vi "drawchart.vi"() -> ()   [LabVIEW 2012]
uses:
  <vilib>/Utility/miscctls.llb/LVDateTimeRec.ctl
  <vilib>/addons/database/Auxilliary.llb/DB Tools Cursor Type.ctl
  <vilib>/addons/database/Connection.llb/DB Tools Open Connec (Path).vi
  <vilib>/addons/database/Connection.llb/Conn Execute.vi
  <vilib>/addons/database/Recordset.llb/Rec Destroy - Connection.vi
  <vilib>/addons/database/_DB Variant To Data/Database Variant To Data.xnode
  <vilib>/addons/database/NI_Database_API.lvlib
panel:
  out "Waveform Graph":i32[](graph)
  out "Array":i32[](array[numeric])
  out "error out":errorcluster
  in  "Cluster":cluster{"rep_date":string, "rep_val":dbl}
  in  "date time rec":T1
  in  "beg_date":string
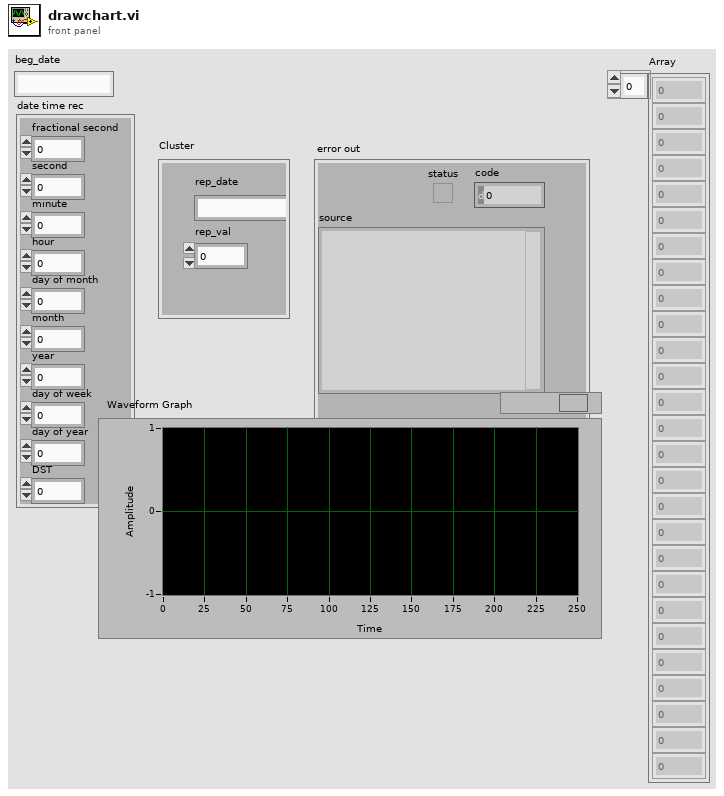
[diagram p1: front panel]
types:
  T1 = typedef "LVDateTimeRec.ctl" = cluster{"fractional second":dbl, "second":i32, "minute":i32, "hour":i32, "day of month":i32, "month":i32, "year":i32, "day of week":i32, "day of year":i32, "DST":i32}
  T2 = typedef "NI_Database_API.lvlib/Conn ObjectReference.ctl" = refnum<k1>
  T3 = typedef "NI_Database_API.lvlib/DB Tools Cursor Type.ctl" = enum16{"forward-only", "keyset", "dynamic", "static"}
  T4 = typedef "NI_Database_API.lvlib/Rec ObjectReference.ctl" = refnum<k1>
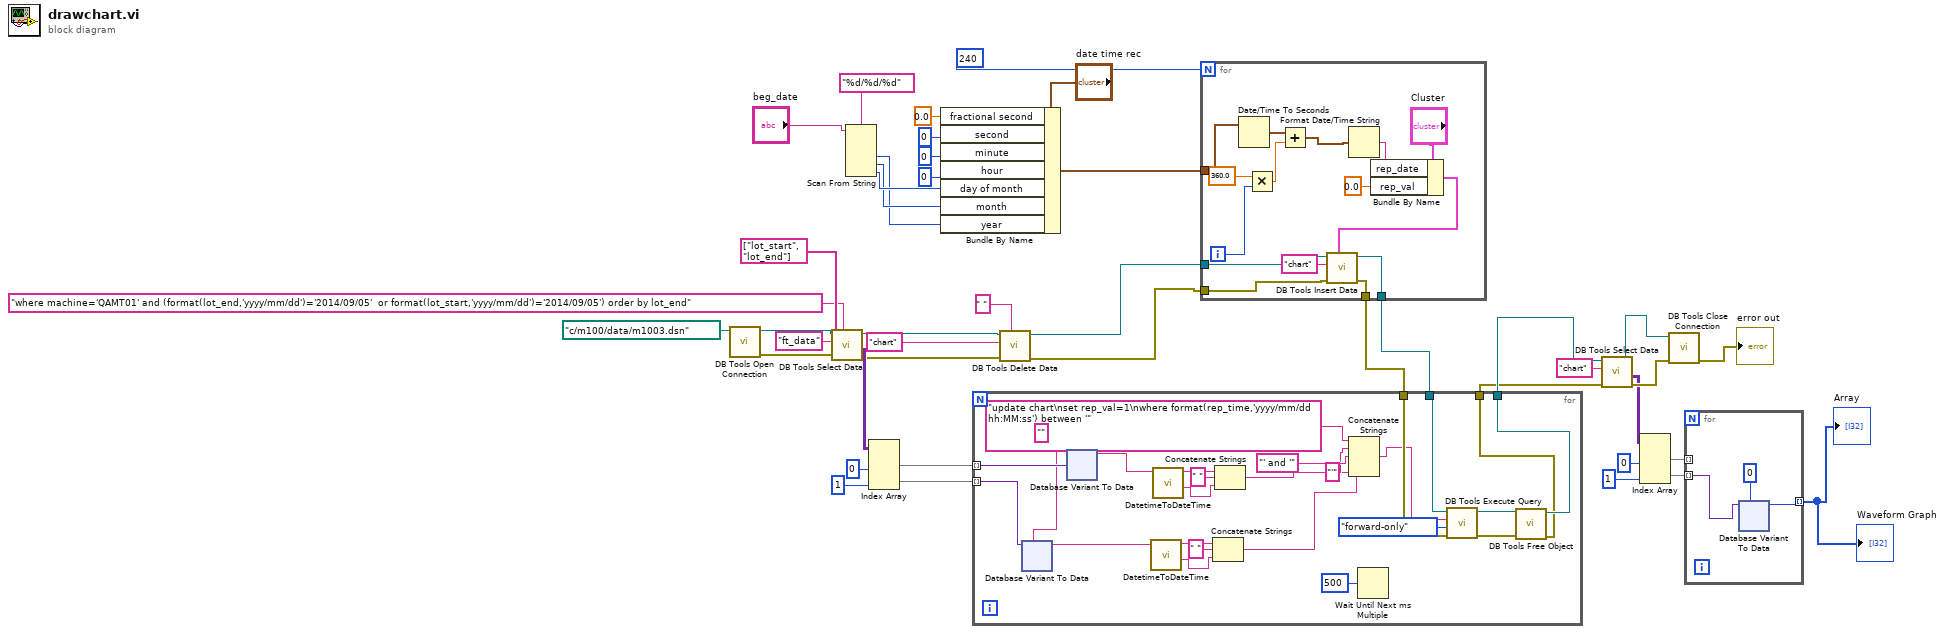
[diagram p0: block diagram]
diagram:
  n1 = call-poly <vilib>:"DB Tools Open Connection.vi"("connection information"=path "c:/m100/data/m1003.dsn") -> ("error out"=w41:errorcluster, "connection reference"=w42:T2)  [unwired: 7 in]
  n2 = call <vilib>:"DB Tools Select Data.vi"("condition"="where machine='QAMT01' and (format(lot_end,'yyyy/mm/dd')='2014/09/05'  or format(lot_start,'yyyy/mm/dd')='2014/09/05') order by lot_end", "error in (no error)"=w41, "columns"=string[] ["lot_start", "lot_end"], "table"="ft_data", "connection reference"=w42) -> ("error out"=w31:errorcluster, "data"=w37:variant[][], "connection reference out"=w32:T2)  [unwired: 1 in]
  n3 = Scan From String(format string="%d/%d/%d", input string="beg_date") -> (output 1=w18:i32, output 2=w19:i32, output 3=w20:i32)  [unwired: 5 in, 3 out]
  n4 = Index Array(array=w37, index (col) #1=0 ("disabled index (col)"), index (col) #2=1 ("index (col)")) -> (element #1=w34:variant[], element #2=w33:variant[])  [unwired: 2 in]
  n5 = Bundle By Name(cluster="date time rec", "fractional second"=0.0, "second"=0, "minute"=0, "hour"=0, "day of month"=w20, "month"=w19, "year"=w18) -> (w17:T1)
  n6 = call <vilib>:"DB Tools Delete Data.vi"("condition"=" ", "error in (no error)"=w31, "table"="chart", "connection reference"=w32) -> ("error out"=w15:errorcluster, "connection reference out"=w16:T2)  [unwired: 6 in]
  n7 = for {
    N: 240 -> [_]
    tunnel: w17 -> [w58]
    tunnel: w16 -> [w49]
    tunnel: w15 -> [w48]
    tunnel: [w45] -> w14
    tunnel: [w44] -> w13
    i -> [w54]
    n8 = Date/Time To Seconds(2:w58) -> (0:w57:timestamp)  [unwired: 1 in]
    n9 = Multiply(x=360.0, y=w54) -> (x*y=w56:dbl)
    n10 = Add(x=w57, y=w56) -> (x+y=w53:timestamp)
    n11 = Format Date/Time String(seconds (now)=w53) -> (date/time string=w52:string)  [unwired: 2 in]
    n12 = Bundle By Name(cluster="Cluster", "rep_date"=w52, "rep_val"=0.0) -> (w46:cluster{"rep_date":string, "rep_val":dbl})
    n13 = call <vilib>:"DB Tools Insert Data.vi"("data"=w46, "error in (no error)"=w48, "table"="chart", "connection reference"=w49) -> ("error out"=w44:errorcluster, "connection reference out"=w45:T2)  [unwired: 6 in]
  }
  n14 = for {
    tunnel: w34 -> [w83] mode=indexing
    tunnel: w33 -> [w82] mode=indexing
    tunnel: w14 -> [w76]
    tunnel: w13 -> [w75]
    tunnel: [w80] -> w11
    tunnel: [w79] -> w9
    w72 = ""
    n15 = xnode "Database Variant To Data"("database variant"=w82, "type"=w72) -> ("data"=w62:string)  [unwired: 1 in, 1 out]
    n16 = xnode "Database Variant To Data"("database variant"=w83, "type"=w72) -> ("data"=w70:string)  [unwired: 1 in, 1 out]
    n17 = call "DatetimeToDateTime.vi"("Datetime string"=w62) -> ("Time string"=w63:string, "Date string"=w65:string)  [unwired: 9 in]
    n18 = call "DatetimeToDateTime.vi"("Datetime string"=w70) -> ("Time string"=w67:string, "Date string"=w69:string)  [unwired: 9 in]
    n19 = Concatenate Strings(w65, " " ("string"), w63) -> (w61:string)
    n20 = Concatenate Strings(w69, " " ("string"), w67) -> (w66:string)
    n21 = Concatenate Strings("update chart\nset rep_val=1\nwhere format(rep_time,'yyyy/mm/dd hh:MM:ss') between '" ("string"), w66, "' and '" ("string"), w61, "'" ("string")) -> (w73:string)
    n22 = Wait Until Next ms Multiple(millisecond multiple=u32 500) -> ()  [unwired: 1 out]
    n23 = call-poly <vilib>:"DB Tools Execute Query.vi"("error in (no error)"=w75, "cursor type"=DB_Tools_Cursor_Type."forward-only", "SQL query"=w73, "connection reference"=w76) -> ("error out"=w77:errorcluster, "recordset reference"=w78:T4)  [unwired: 4 in]
    n24 = call-poly <vilib>:"DB Tools Free Object.vi"("error in (no error)"=w77, "recordset reference"=w78) -> ("error out"=w79:errorcluster, "connection reference"=w80:T2)  [unwired: 8 in]
  }
  n25 = call <vilib>:"DB Tools Select Data.vi"("error in (no error)"=w9, "table"="chart", "connection reference"=w11) -> ("error out"=w8:errorcluster, "data"=w6:variant[][], "connection reference out"=w10:T2)  [unwired: 3 in]
  n26 = Index Array(array=w6, index (col) #1=0 ("disabled index (col)"), index (col) #2=1 ("index (col)")) -> (element #1=w3:variant[], element #2=w2:variant[])  [unwired: 2 in]
  n27 = call <vilib>:"DB Tools Close Connection.vi"("error in (no error)"=w8, "connection reference"=w10) -> ("error out"=→"error out":errorcluster)  [unwired: 5 in]
  n28 = for {
    tunnel: w3 -> [_] mode=indexing
    tunnel: w2 -> [w150] mode=indexing
    tunnel: [w148] -> w1 mode=indexing
    n29 = xnode "Database Variant To Data"("database variant"=w150, "type"=0) -> ("data"=w148:i32)  [unwired: 1 in, 1 out]
  }
  "Array" <- w1
  "Waveform Graph" <- w1
